vi "Read local path.vi"(8 "error in":errorcluster, 11 "Shared Library Module editor node in":refnum<class "Shared Library Module editor node.lvclass">) -> (0 "error out":errorcluster, 2 "local path":path, 3 "Shared Library Module editor node out":refnum<class "Shared Library Module editor node.lvclass">)   [LabVIEW 2013, in "Shared Library Module editor node.lvclass"]
uses:
  Shared Library Module editor node.lvclass
  Shared Library Module editor node.lvclass/Shared Library Module editor node.ctl
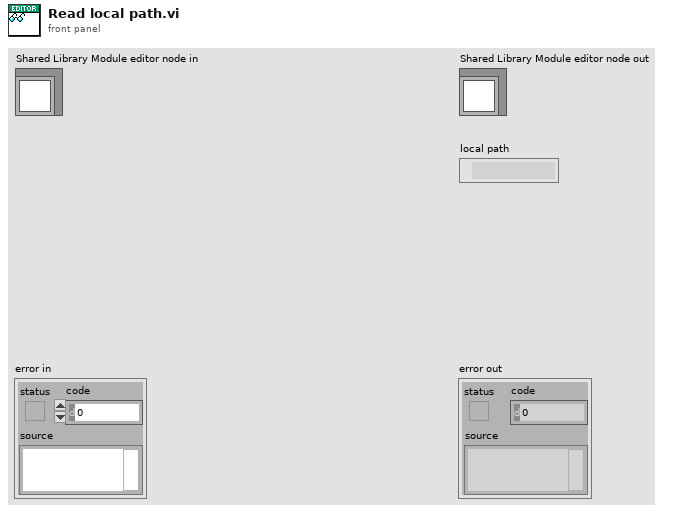
[diagram p1: front panel]
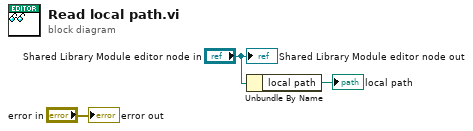
[diagram p0: block diagram]
diagram:
  n1 = Unbundle By Name("Shared Library Module editor node in") -> ("local path"=→"local path":path)
  "error out" <- "error in"
  "Shared Library Module editor node out" <- "Shared Library Module editor node in"
